vi "CAPFM-Initialize.vi"(0 "Expt State":T28, 5 "CAPFM Params":T29, 11 "error in (no error)":errorcluster) -> (4 "Runtime":T1, 6 "StimChans":T3[](xcontrol), 10 "Intervals (ms)":dbl[](array[numeric]), 14 "Analysis":T2, 15 "error out":errorcluster)   [LabVIEW 2020]
uses:
  Typedefs/CAPFM-All Params.ctl
  epl-vi-lib/Utility VIs/Type Defs/Left-Right ring.ctl
  Typedefs/CAPFM-Probe Params.ctl
  Typedefs/CAPFM-Masker Params.ctl
  Typedefs/CAPFM-Seq Params.ctl
  Typedefs/CAPFM-Timing Params.ctl
  Typedefs/CAPFM-Response Params.ctl
  CFTS Main Panel SubVIs/CFTS-Experiment State.ctl
  epl-vi-lib/Signal Synthesis VIs/Controls/Multichannel (Full)/Multichannel (Full).xctl
  Typedefs/CAPFM-Analysis State.ctl
  Typedefs/CAPFM-Runtime Data.ctl
  <vilib>/Analysis/3filter.llb/Filter Passband Type.ctl
  <vilib>/Analysis/4window.llb/windowTd.ctl
  <vilib>/Analysis/1siggen.llb/Riffle Array (DBL) (obs 2012).vi
  epl-vi-lib/Signal Synthesis VIs/Top Level VIs/Stimulus-Initialize (full array).vi
  <vilib>/Analysis/NI_AALBase.lvlib
  <vilib>/Analysis/NI_AALPro.lvlib
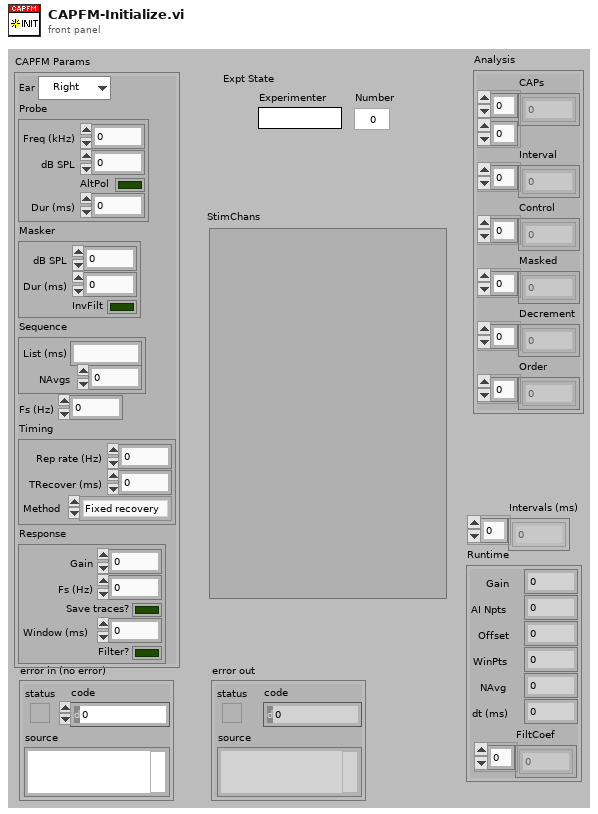
[diagram p1: front panel]
types:
  T1 = typedef "CAPFM-Runtime Data.ctl" = cluster{"Offset":i32, "AI Npts":i32, "Gain":dbl, "WinPts":i32, "NAvg":i32, "dt (ms)":dbl, "FiltCoef":dbl[]}
  T2 = typedef "CAPFM-Analysis State.ctl" = cluster{"CAPs":dbl[][], "Interval":dbl[], "Control":dbl[], "Masked":dbl[], "Decrement":dbl[], "Order":i32[]}
  T3 = typedef "Stimulus Channel (Full).xctl/Full Stimulus Channel Data.ctl" = cluster{"Waveform":T4, "Filter":T21, "Burst":T23, "Level":T24, "Name":string, "Advanced":T26, "SAM":T27}
  T4 = typedef "Waveform XCtl.xctl/Waveform Data.ctl" = cluster{"Type":T5, "Tone":T6, "Pulse Train":T7, "Noise":T10, "File":T11, "FMSweep":T12, "Chirp Train":T13, "Complex Tone":cluster{"Params":T15, "Data":T17}, "Moving Ripple":T18}
  T5 = typedef "Waveform Enum.ctl" = enum16{"OFF", "Tone", "Noise", "Pulse Train", "File", "FM Sweep", "Chirp Train", "Complex Tone", "FM Tone", "Moving Ripple"}
  T6 = typedef "Tone Params.ctl" = cluster{"Frequency (kHz)":dbl, "Last Freq":dbl, "Last Phase":dbl}
  T7 = typedef "Pulse Train Params.ctl" = cluster{"Pulse width (us)":dbl, "Pulse rate (Hz)":dbl, "Gap (ms)":dbl, "Polarity":T8, "PT State":T9, "Asynch":bool}
  T8 = typedef "Pulse Polarity.ctl" = enum16{"POS", "NEG", "POS-NEG", "NEG-POS"}
  T9 = typedef "PT-Continuous State.ctl" = cluster{"Template":dbl[], "Nperiod":i32, "Index":i32, "Pulse Rate (Hz)":dbl, "Phase (cycles)":dbl, "Noff":i32}
  T10 = typedef "Noise Params.ctl" = cluster{"InvFilt":bool, "Noise":dbl[], "CurPt":i32, "Aweight":bool, "Seed":i32, "afile":path}
  T11 = typedef "StimFile-Params.ctl" = cluster{"Filename":path, "Signal":dbl[], "Channel":i32, "stream":bool, "offset":i32, "nreps":i32, "loops":i32, "Randomize":bool, "order":i32[], "Seed":i32, "Tokens":i32}
  T12 = typedef "FM Sweep Params.ctl" = cluster{"Rate (oct/s)":dbl, "Fmin (Hz)":dbl, "Fmax (Hz)":dbl, "Ramp (ms)":dbl, "Linear":bool}
  T13 = typedef "Chirp Train.ctl" = cluster{"Params":T14, "Data":cluster{"WF":dbl[]}}
  T14 = typedef "Chirp Train Params.ctl" = cluster{"Fmin (kHz)":dbl, "Fmax (kHz)":dbl, "Compensate":bool, "Duration (ms)":dbl}
  T15 = typedef "CT-Params.ctl" = cluster{"F0 (Hz)":dbl, "Band":cluster{"Flow (Hz)":dbl, "Fhigh (Hz)":dbl}, "Phase":T16, "Min F0 (Hz)":dbl, "Max F0 (Hz)":dbl, "ContinRandPhase":bool, "Max peak factor":dbl, "Max mod depth":dbl, "MinHarmNum":i32, "MaxHarmNum":i32, "Level Mode":enum16{"per component", "overall rms"}, "% jitter":dbl}
  T16 = typedef "CT-Phase Enum.ctl" = enum16{"Cosine", "Random", "Alternating"}
  T17 = typedef "CT-Runtime Data.ctl" = cluster{"Ncomp":i32, "MinHarm":i32, "Phase":dbl[], "Amplitude":dbl[], "Npts/frame":i32, "Last F0":dbl, "Fmin":dbl, "Fmax":dbl, "Lslope":dbl, "randphase":bool, "overall rms":bool, "fmult":dbl[], "jittered":bool}
  T18 = typedef "Moving Ripple.ctl" = cluster{"Params":T19, "Data":T20}
  T19 = typedef "Moving Ripple.Params.ctl" = cluster{"Fmin":dbl, "Fmax":dbl, "Density":dbl, "Velocity":dbl, "Depth":dbl, "Phase":dbl, "Comp/oct":i32}
  T20 = typedef "Moving Ripple.Data.ctl" = cluster{"Freq":dbl[], "A":dbl[], "phase":dbl[], "Phase":dbl}
  T21 = typedef "Advanced Filter XCtl.xctl/Filter Data.ctl" = cluster{"Type":enum16{"Lowpass", "Highpass", "Bandpass", "Bandstop", "OFF"}, "CF (kHz)":dbl, "BW (kHz)":dbl, "Cascade":bool, "Quadrature":bool, "Scale Factor":dbl, "Stages":cluster{"IIR Filter":cluster{"filter structure":enum32{"IIR 2nd Order", "IIR 4th Order"}, "Reverse Coefficients":dbl[], "Forward Coefficients":dbl[]}, "State":dbl[]}[], "Class":enum16{"Elliptic", "Butterworth"}, "Order":i32, "BWUnits":T22}
  T22 = typedef "Filter-Bandwidth Units.ctl" = enum16{"Linear", "Octaves", "Min-Max"}
  T23 = typedef "Burst Control.xctl/Burst Data.ctl" = cluster{"Active":bool, "Delay (ms)":dbl, "Duration (ms)":dbl, "Ramp (ms)":dbl, "Rate (Hz)":dbl, "Trepeat (ms)":dbl, "Repeat":bool}
  T24 = typedef "Level XCtl.xctl/Level Data.ctl" = cluster{"Level":dbl, "Units":T25, "Max":dbl, "Multiplier":dbl, "Cal File":path, "Cal":cluster{"Freq (Hz)":dbl[], "Mag (dB SPL)":dbl[], "Phase (deg)":dbl[]}}
  T25 = typedef "Level Units.ctl" = enum16{"dB atten", "dB SPL", "dB re 1 Vrms", "dB V/Hz½", "mW", "dB HL", "Volts", "dB mW"}
  T26 = typedef "Advanced Stimulus Options.xctl/Advanced Stimulus Options.ctl" = cluster{"Rep Mask":string, "AltPol":bool, "Var":string, "Expr":string, "Persist":bool}
  T27 = typedef "SAM Params.ctl" = cluster{"Active":bool, "Frequency (Hz)":dbl, "Depth":dbl, "Init Phase (cycles)":dbl, "phase (degrees)":dbl, "Asynch":bool}
  T28 = typedef "CFTS-Experiment State.ctl" = cluster{"Experimenter":string, "Number":u32, "Right":string, "Left":string, "Data Folder":path, "State File":path, "Version Info":string, "End Exposure Time":dbl, "Exposure Duration":string, "Run #":cluster{"CAP":i16, "ABR":i16, "DP":i16, "VsEP":i16, "MeasSeq":i16, "SubSeq":i16, "SFOAE":i16}}
  T29 = typedef "CAPFM-All Params.ctl" = cluster{"Ear":T30, "Probe":T31, "Masker":T32, "Sequence":T33, "Fs (Hz)":dbl, "Timing":T34, "Response":T35}
  T30 = typedef "Left-Right ring.ctl" = enum16{"Right", "Left"}
  T31 = typedef "CAPFM-Probe Params.ctl" = cluster{"Freq (kHz)":dbl, "dB SPL":dbl, "AltPol":bool, "Dur (ms)":dbl}
  T32 = typedef "CAPFM-Masker Params.ctl" = cluster{"dB SPL":dbl, "Dur (ms)":dbl, "InvFilt":bool}
  T33 = typedef "CAPFM-Seq Params.ctl" = cluster{"List (ms)":string, "NAvgs":i32}
  T34 = typedef "CAPFM-Timing Params.ctl" = cluster{"Rep rate (Hz)":dbl, "TRecover (ms)":dbl, "Method":enum16{"Fixed recovery", "Fixed rep rate"}}
  T35 = typedef "CAPFM-Response Params.ctl" = cluster{"Gain":dbl, "Fs (Hz)":dbl, "Save traces?":bool, "Window (ms)":dbl, "Filter?":bool}
  T36 = typedef "NI_AALBase.lvlib/Filter Passband Type.ctl" = enum32{"Lowpass", "Highpass", "Bandpass", "Bandstop"}
  T37 = typedef "NI_AALPro.lvlib/windowTd.ctl" = u32
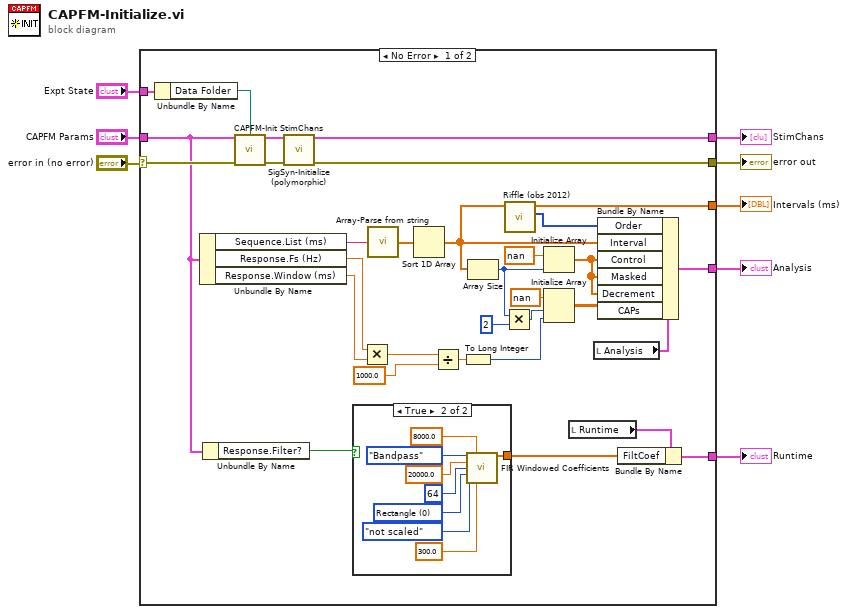
[diagram p0: block diagram]
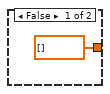
[diagram p2: hidden frame]
diagram:
  n1 = case shown="No Error" "error in (no error)" {
    selector: "error in (no error)" -> [w40 w50]
    tunnel: [w36 w50] -> w7
    tunnel: "CAPFM Params" -> [w13 _]
    tunnel: "Expt State" -> [w39 _]
    tunnel: [w34 _] -> w4
    tunnel: [w28 _] -> w3
    tunnel: [w31 _] -> w2
    tunnel: [w11 _] -> w1
    frame No Error {
      n2 = Unbundle By Name(w39) -> ("Data Folder"=w38:path)
      n3 = Unbundle By Name(w13) -> ("Sequence.List (ms)"=w16:string, "Response.Fs (Hz)"=w23:dbl, "Response.Window (ms)"=w22:dbl)
      n4 = Unbundle By Name(w13) -> ("Response.Filter?"=w10:bool)
      n5 = call "CAPFM-Init StimChans.vi"("Params"=w13, "Data Folder"=w38, "error in (no error)"=w40) -> ("StimChans"=w37:T3[], "error out"=w35:errorcluster)  [unwired: 11 in]
      n6 = call-poly "SigSyn-Initialize (polymorphic).vi"("StimChans"=w37, "error in (no error)"=w35) -> ("StimChans Out"=w34:T3[], "error out"=w36:errorcluster)  [unwired: 11 in, 1 out]
      n7 = case shown="True" w10 {
        tunnel: [dbl[] [] ("FIR Windowed Coefficients") w42] -> w9
        frame False {
        }
        frame True {
          w46 = T37 0 items=["Rectangle"=0, "Hanning"=1, "Hamming"=2, "Blackman-Harris"=3, "Exact Blackman"=4, "Blackman"=5, "Flat Top"=6, "4 Term B-Harris "=7, "7 Term B-Harris"=8, "Low Sidelobe"=9, "Blackman Nuttall"=11, "Triangle"=30, "Bartlett-Hanning"=31, "Bohman"=32, "Parzen"=33, "Welch"=34, "Kaiser"=60, "Dolph-Chebyshev"=61, "Gaussian"=62] ("window")
          n8 = call <vilib>:"FIR Windowed Coefficients.vi"("filter type"=Filter_Passband_Type."Bandpass", "high cutoff freq: fh"=8000.0, "sampling freq: fs"=20000.0, "taps"=64, "window"=w46, "option"=enum32{"not scaled", "scaled"}."not scaled", "low cutoff freq: fl"=300.0) -> ("FIR Windowed Coefficients"=w42:dbl[])  [unwired: 7 in, 1 out]
        }
      }
      n9 = Multiply(x=w23, y=w22) -> (x*y=w26:dbl)
      n10 = call "Array-Parse from string.vi"("String"=w16) -> ("Array"=w15:dbl[])  [unwired: 13 in, 1 out]
      n11 = Sort 1D Array(array=w15) -> (sorted array=w14:dbl[])
      n12 = Divide(x=w26, y=1000.0) -> (x/y=w24:dbl)
      n13 = To Long Integer(number=w24) -> (32bit integer=w21:i32)
      n14 = Array Size(array=w14) -> (size(s)=w18:i32)
      n15 = Multiply(x=w18, y=2) -> (x*y=w19:i32)
      n16 = call-poly <vilib>:"Riffle (obs 2012).vi"("X"=w14) -> ("Riffled Index"=w32:i32[], "Riffled {X}"=w28:dbl[])  [unwired: 8 in, 1 out]
      n17 = Initialize Array(nan ("element"), w18) -> (w29:dbl[])
      n18 = Initialize Array(nan ("element"), w19, w21) -> (w20:dbl[][])
      n19 = local read "Runtime"() -> (w12:T1)
      n20 = local read "Analysis"() -> (w33:T2)
      n21 = Bundle By Name(cluster=w33, "Order"=w32, "Interval"=w14, "Control"=w29, "Masked"=w29, "Decrement"=w29, "CAPs"=w20) -> (w31:T2)
      n22 = Bundle By Name(cluster=w12, "FiltCoef"=w9) -> (w11:T1)
    }
    frame Error {
    }
  }
  "error out" <- w7
  "StimChans" <- w4
  "Analysis" <- w2
  "Runtime" <- w1
  "Intervals (ms)" <- w3
